vi "labview_f3.vi"() -> ()   [LabVIEW 2015]
panel:
  out "Boolean":bool
  out "Meter":i32(knob) scale=1.0..6.0
  out "Numeric":i32
  in  "OK Button":bool
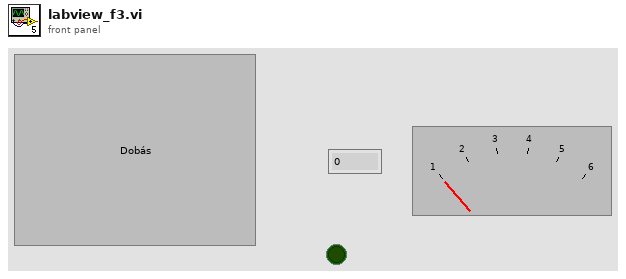
[diagram p1: front panel]
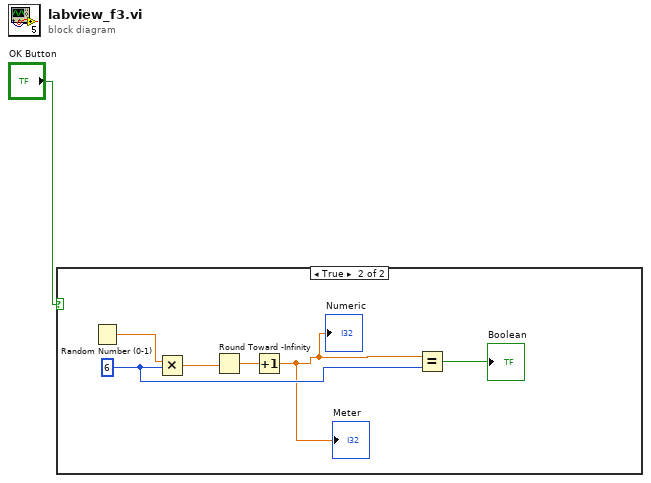
[diagram p0: block diagram]
diagram:
  n1 = case shown="True" "OK Button" {
    frame False {
    }
    frame True {
      w4 = 6
      n2 = Random Number (0-1) ("Random Number (1-6)")() -> (number: 0 to 1=w5:dbl)
      n3 = Multiply(x=w5, y=w4) -> (x*y=w6:dbl)
      n4 = Round Toward -Infinity(1:w6) -> (0:w7:dbl)
      n5 = Increment(x=w7) -> (x+1=w3:dbl)
      "Numeric" <- w3
      "Meter" <- w3
      n6 = Equal?(x=w3, y=w4) -> (x = y?=→"Boolean":bool)
    }
  }
